vi "Log.vi"(8 "error in (no error)":errorcluster, 10 "tdms file":refnum<k34>, 11 "Acquired Result in":refnum<class "Acquired Result.lvclass">) -> (0 "error out":errorcluster, 2 "tdms file out":refnum<k34>, 3 "Acquired Result out":refnum<class "Acquired Result.lvclass">)   [LabVIEW 2016, in "Acquired Result.lvclass"]
uses:
  Acquired Result.lvclass
  Acquired Result.lvclass/Acquired Result.ctl
  Read Group.vi
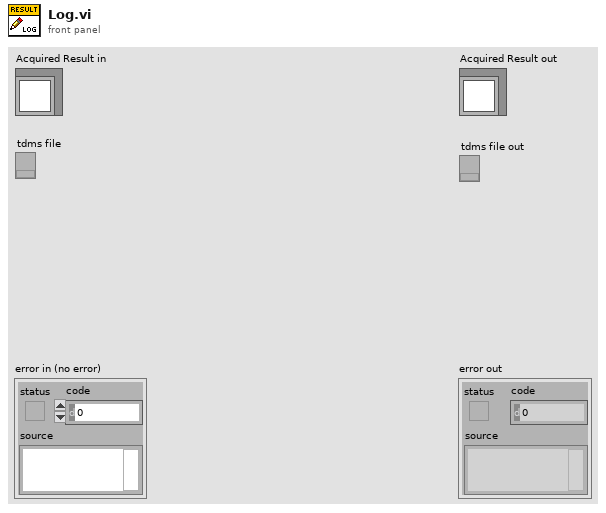
[diagram p1: front panel]
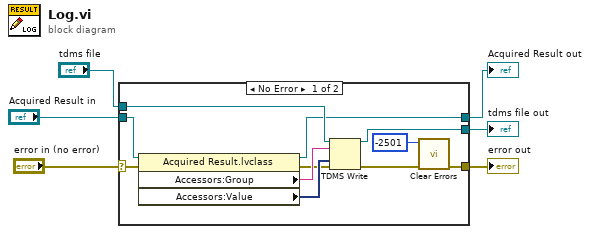
[diagram p0: block diagram]
diagram:
  n1 = case shown="No Error" "error in (no error)" {
    selector: "error in (no error)" -> [w9 w18]
    tunnel: "Acquired Result in" -> [w17 w20]
    tunnel: "tdms file" -> [w16 w19]
    tunnel: [w15 w19] -> w4
    tunnel: [w14 w20] -> w3
    tunnel: [w8 w18] -> w2
    frame No Error {
      n2 = property class="Acquired Result.lvclass"(reference=w17, error in=w9) -> (reference out=w14:refnum<class "Acquired Result.lvclass">, error out=w10:errorcluster, "Accessors:Group"=w13:string, "Accessors:Value"=w12:dynamicdata)
      n3 = TDMS Write(0:w16, 5:w13, 9:w12, 11:w10) -> (4:w15:refnum<k34>, 15:w11:errorcluster)  [unwired: 2 in, 2 out]
      n4 = call <vilib>:"Clear Errors.vi"("error in (no error)"=w11, "specific error code to clear (0: all)"=-2501) -> ("error out"=w8:errorcluster)  [unwired: 4 in, 1 out]
    }
    frame Error {
    }
  }
  "error out" <- w2
  "Acquired Result out" <- w3
  "tdms file out" <- w4
